vi "ParseStudicaChannel.vi"(11 "Array":u8[](array[numeric])) -> (1 "ButtonsAndOther":u8[](array[numeric]), 2 "Sensors":sgl[](array[numeric]), 3 "Encs":i32[](array[numeric]))   [LabVIEW 2019]
panel:
  out "Yaw":sgl
  out "Analog":u16[](array[numeric])
  out "Us":sgl[](array[numeric])
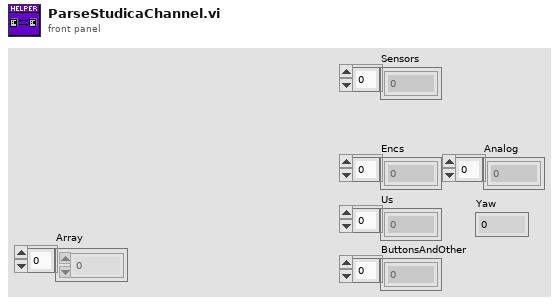
[diagram p1: front panel]
types:
  T1 = enum16{"big-endian, network order", "native, host order", "little-endian"}
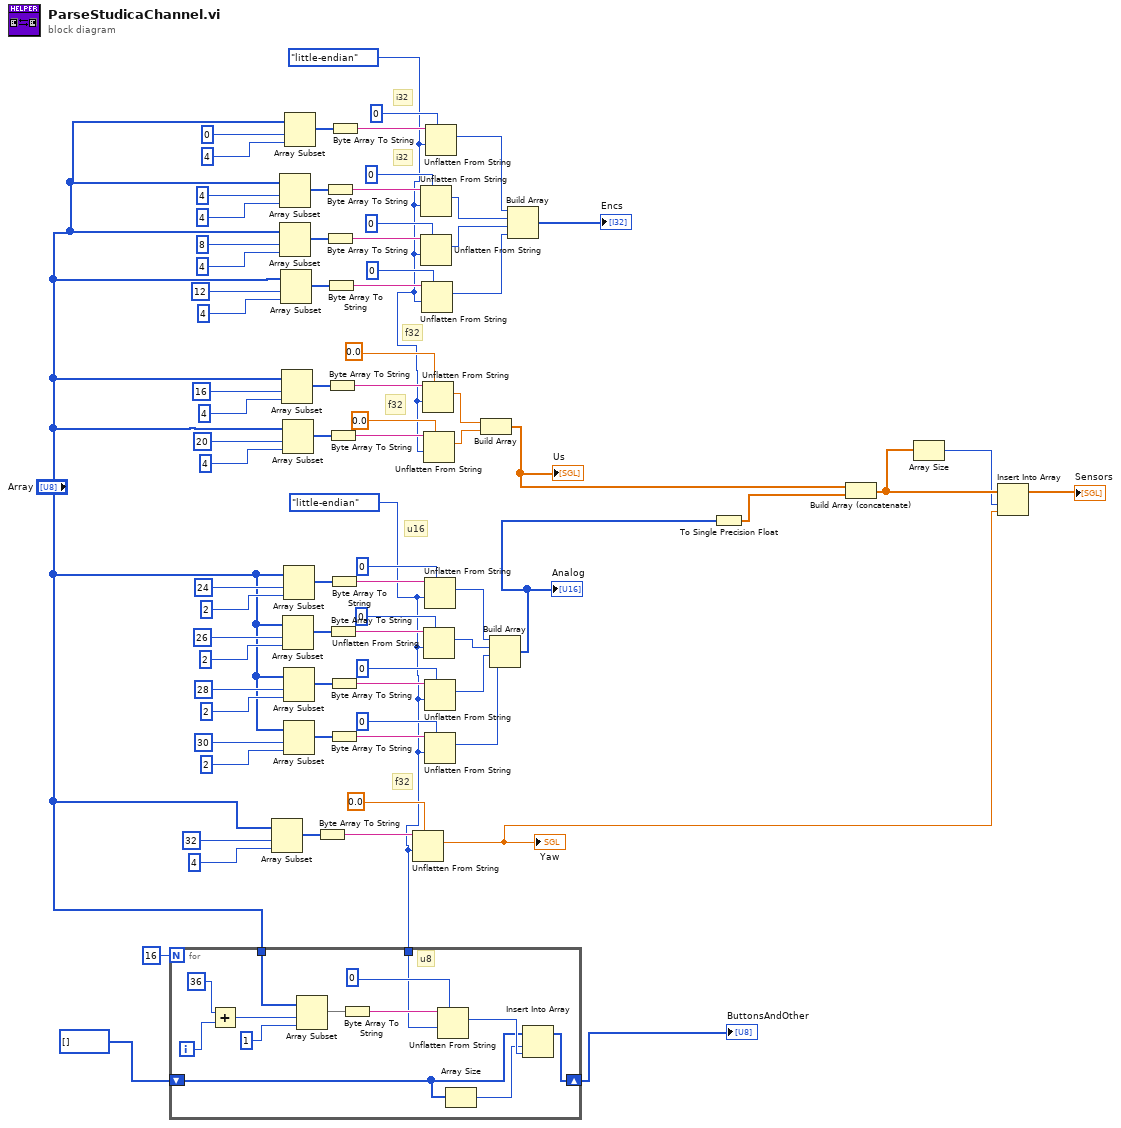
[diagram p0: block diagram]
diagram:
  w2 = T1."little-endian" ("byte order (0:big-endian, network order)")
  w1 = T1."little-endian" ("byte order (0:big-endian, network order)")
  # "f32"
  # "i32"
  # "f32"
  # "u16"
  # "f32"
  # "i32"
  n1 = for {
    N: 16 -> [_]
    tunnel: "Array" -> [w89]
    shift-right: [w84] -> w3
    shift-left: u8[] [] -> [w82]
    tunnel: w1 -> [w80]
    i -> [w86]
    # "u8"
    n2 = Add(x=36 ("index"), y=w86) -> (x+y=w88:i32)
    n3 = Array Subset(array=w89, index=w88, length=1) -> (w91:u8[])
    n4 = Byte Array To String(unsigned byte array=w91) -> (string=w90:string)
    n5 = Unflatten From String(type=u8 0, binary string=w90, byte order (0:big-endian, network order)=w80) -> (value=w83:u8)  [unwired: 2 in, 2 out]
    n6 = Array Size(array=w82) -> (size(s)=w81:i32)
    n7 = Insert Into Array(array=w82, index=w81, new element=w83) -> (w84:u8[])
  }
  "ButtonsAndOther" <- w3
  n8 = Array Subset(array="Array", index=32, length=4) -> (w65:u8[])
  n9 = Array Subset(array="Array", index=4, length=4) -> (w54:u8[])
  n10 = Array Subset(array="Array", index=8, length=4) -> (w49:u8[])
  n11 = Array Subset(array="Array", index=12, length=4) -> (w44:u8[])
  n12 = Array Subset(array="Array", index=16, length=4) -> (w73:u8[])
  n13 = Array Subset(array="Array", index=20, length=4) -> (w33:u8[])
  n14 = Array Subset(array="Array", index=26, length=2) -> (w24:u8[])
  n15 = Array Subset(array="Array", index=24, length=2) -> (w69:u8[])
  n16 = Array Subset(array="Array", index=28, length=2) -> (w19:u8[])
  n17 = Array Subset(array="Array", index=30, length=2) -> (w14:u8[])
  n18 = Array Subset(array="Array", index=0, length=4) -> (w77:u8[])
  n19 = Byte Array To String(unsigned byte array=w65) -> (string=w64:string)
  n20 = Byte Array To String(unsigned byte array=w54) -> (string=w53:string)
  n21 = Byte Array To String(unsigned byte array=w49) -> (string=w48:string)
  n22 = Byte Array To String(unsigned byte array=w44) -> (string=w43:string)
  n23 = Byte Array To String(unsigned byte array=w73) -> (string=w72:string)
  n24 = Byte Array To String(unsigned byte array=w33) -> (string=w32:string)
  n25 = Byte Array To String(unsigned byte array=w24) -> (string=w23:string)
  n26 = Byte Array To String(unsigned byte array=w69) -> (string=w68:string)
  n27 = Byte Array To String(unsigned byte array=w19) -> (string=w18:string)
  n28 = Byte Array To String(unsigned byte array=w14) -> (string=w13:string)
  n29 = Byte Array To String(unsigned byte array=w77) -> (string=w76:string)
  n30 = Unflatten From String(type=sgl 0.0, binary string=w64, byte order (0:big-endian, network order)=w1) -> (value=w60:sgl)  [unwired: 2 in, 2 out]
  "Yaw" <- w60
  n31 = Unflatten From String(type=0, binary string=w53, byte order (0:big-endian, network order)=w2) -> (value=w40:i32)  [unwired: 2 in, 2 out]
  n32 = Unflatten From String(type=0, binary string=w48, byte order (0:big-endian, network order)=w2) -> (value=w39:i32)  [unwired: 2 in, 2 out]
  n33 = Unflatten From String(type=0, binary string=w43, byte order (0:big-endian, network order)=w2) -> (value=w38:i32)  [unwired: 2 in, 2 out]
  n34 = Unflatten From String(type=sgl 0.0, binary string=w72, byte order (0:big-endian, network order)=w2) -> (value=w30:sgl)  [unwired: 2 in, 2 out]
  n35 = Unflatten From String(type=sgl 0.0, binary string=w32, byte order (0:big-endian, network order)=w2) -> (value=w29:sgl)  [unwired: 2 in, 2 out]
  n36 = Unflatten From String(type=u16 0, binary string=w23, byte order (0:big-endian, network order)=w1) -> (value=w10:u16)  [unwired: 2 in, 2 out]
  n37 = Unflatten From String(type=u16 0, binary string=w68, byte order (0:big-endian, network order)=w1) -> (value=w11:u16)  [unwired: 2 in, 2 out]
  n38 = Unflatten From String(type=u16 0, binary string=w18, byte order (0:big-endian, network order)=w1) -> (value=w9:u16)  [unwired: 2 in, 2 out]
  n39 = Unflatten From String(type=u16 0, binary string=w13, byte order (0:big-endian, network order)=w1) -> (value=w8:u16)  [unwired: 2 in, 2 out]
  n40 = Unflatten From String(type=0, binary string=w76, byte order (0:big-endian, network order)=w2) -> (value=w41:i32)  [unwired: 2 in, 2 out]
  n41 = Build Array(w30, w29) -> (w28:sgl[])
  "Us" <- w28
  n42 = Build Array(w11, w10, w9, w8) -> (w7:u16[])
  "Analog" <- w7
  n43 = Build Array(w41, w40, w39, w38) -> (→"Encs":i32[])
  n44 = To Single Precision Float(number=w7) -> (single precision float=w62:sgl[])
  n45 = Build Array (concatenate)(w28, w62) -> (w61:sgl[])
  n46 = Array Size(array=w61) -> (size(s)=w59:i32)
  n47 = Insert Into Array(array=w61, index=w59, new element=w60) -> (→"Sensors":sgl[])
